vi "Initialize.vi"(5 "instance":u8) -> (4 "subsystem":refnum<class "Single Address Space Collection.lvclass">, 6 "AddressSpace":refnum<class "AddressSpace.lvclass">)   [LabVIEW 2017, in "SVPWM.lvlib" / "AddressSpace.lvclass"]
uses:
  AddressSpace.lvclass
  <instrlib>/_niInstr/Instruction Framework/v1/FPGA/Helper Classes/Single Address Space Collection/Single Address Space Collection.lvclass
  C:/Program Files (x86)/National Instruments/LabVIEW 2017/instr.lib/_niInstr/Instruction Framework/v1/FPGA/Interfaces/Address Space/Address Space.lvclass
  AddressSpace.lvclass/AddressSpace.ctl
  <vilib>/rvi/DataTransferAndStorage/Container/Common/niFpgaContainerGetUniqueNameForEmu.vi
  <vilib>/rvi/DataTransferAndStorage/Container/Common/niFpgaContainerSetEmuInfo.vi
  <vilib>/rvi/eio/common/nirviEmuReportErrorAndStop.vi
  <vilib>/rvi/LocalResourceManager/LocalResourceManager.xnode
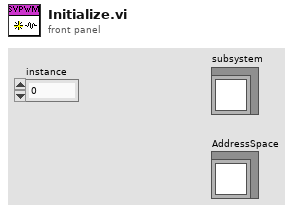
[diagram p1: front panel]
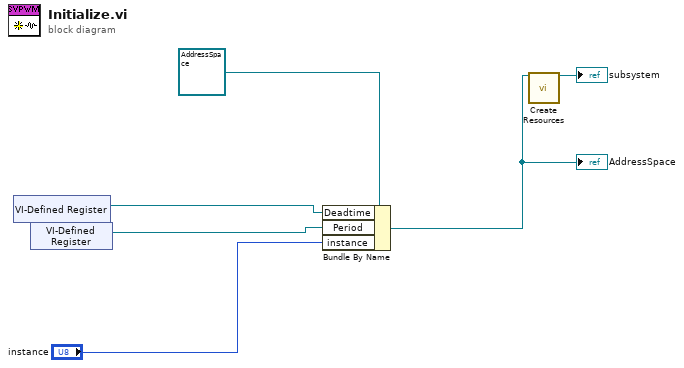
[diagram p0: block diagram]
diagram:
  n1 = xnode "VI-Defined Register"() -> ("Register Out"=w1:refnum<k21>)
  n2 = xnode "VI-Defined Register"() -> ("Register Out"=w2:refnum<k21>)
  n3 = Bundle By Name(cluster=refnum<class "AddressSpace.lvclass"> refnum ("SVPWM.lvlib:AddressSpace.lvclass"), "Deadtime"=w1, "Period"=w2, "instance"="instance") -> (w3:refnum<class "AddressSpace.lvclass">)
  "AddressSpace" <- w3
  n4 = call <instrlib>:"Create Resources.vi"("address space"=w3) -> ("single address space collection"=→"subsystem":refnum<class "Single Address Space Collection.lvclass">)  [unwired: 14 in]
